vi "Generate All Library HTML Documentation.vi"(6 "Requirement":string="Labstache", 7 "Destination":path=path "", 8 "Error In":errorcluster, 11 "Source In":path=path "") -> (0 "Error Out":errorcluster, 3 "Source Out":path)   [LabVIEW 2018, in "Scripts.lvlib"]
uses:
  Scripts.lvlib
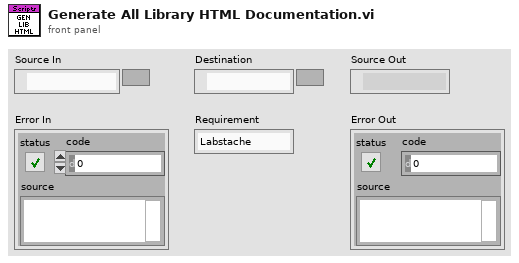
[diagram p1: front panel]
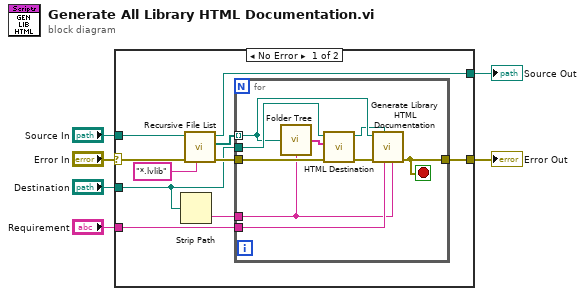
[diagram p0: block diagram]
diagram:
  n1 = case shown="No Error" "Error In" {
    selector: "Error In" -> [w10 w27]
    tunnel: "Requirement" -> [w13 _]
    tunnel: [w12 w27] -> w5
    tunnel: "Destination" -> [w8 _]
    tunnel: "Source In" -> [w11 w26]
    tunnel: [w9 w26] -> w1
    frame No Error {
      n2 = Strip Path(path=w8) -> (name=w7:string)  [unwired: 1 out]
      n3 = call <vilib>:"Recursive File List.vi"("pattern"="*.lvlib", "error in (no error)"=w10, "Folder Path"=w11) -> ("error out"=w14:errorcluster, "All Files in Dir"=w15:path[], "dup Folder Path"=w9:path)  [unwired: 4 in, 2 out]
      n4 = for {
        tunnel: w15 -> [w20] mode=indexing
        tunnel: w14 -> [w22]
        tunnel: [w25] -> w12
        tunnel: w13 -> [w18]
        tunnel: w7 -> [w17]
        tunnel: w8 -> [w23]
        stop <- w25 stop-if-true
        n5 = call "Folder Tree.vi"("File"=w20, "Root Folder Name"=w17) -> ("Hierarchy Folders"=w24:string[])
        n6 = call "HTML Destination.vi"("Error In"=w22, "Hierarchy Folders"=w24, "Root Destination"=w23) -> ("Error Out"=w21:errorcluster, "HTML Destination"=w19:path)  [unwired: 7 in]
        n7 = call "Generate Library HTML Documentation.vi"("Root Folder Name"=w17, "Requirement"=w18, "Destination"=w19, "Error In"=w21, "Library File"=w20) -> ("Error Out"=w25:errorcluster)  [unwired: 6 in]
      }
    }
    frame Error {
    }
  }
  "Error Out" <- w5
  "Source Out" <- w1
